vi "XDataNode8_6To8_5.vi"(10 "Version-State Cluster In":T1, 11 "XRef":refnum<vi>) -> (0 "Custom Label":string, 1 "Custom Warning To Issue":string, 2 "Version-State Cluster Out":T1, 3 "Action":T2)   [LabVIEW 2020]
uses:
  <vilib>/XSFPSupport/SFPChangeStateAction.ctl
  <vilib>/XNodeSupport/XNodeVersion.ctl
  <vilib>/XNodeSupport/XNodeUShort.ctl
  <vilib>/Platform/TimedLoop/XDataNode/XDataNode.ctl
  <vilib>/Platform/TimedLoop/XDataNode/timing_clust.ctl
  <vilib>/Platform/TimedLoop/XDataNode/nitl_modes.ctl
  <vilib>/Platform/TimedLoop/XDataNode/wakeup.ctl
  <vilib>/Platform/TimedLoop/XDataNode/TermInfo.ctl
  <vilib>/Platform/TimedLoop/XDataNode/nitl_TargetSpecificData.ctl
  <vilib>/Platform/TimedLoop/XDataNode/DN_Type.ctl
  <vilib>/Platform/TimedLoop/XDataNode/XDataNode8_5_0_1.ctl
  <vilib>/XSFPSupport/NI_XSFPSupport.lvlib
  <vilib>/XNodeSupport/NI_XNodeSupport.lvlib
  <vilib>/Platform/TimedLoop/XDataNode/XDataNode.xnode
  <vilib>/Platform/TimedLoop/XDataNode/XDNodeRunTimeDep.lvlib
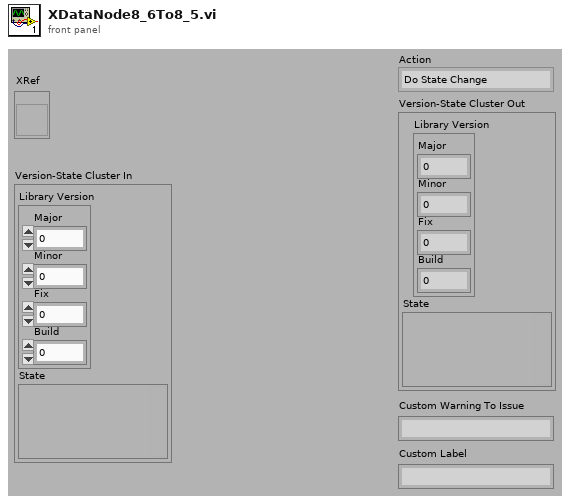
[diagram p1: front panel]
types:
  T1 = cluster{"Library Version":cluster{"Major":u16, "Minor":u16, "Fix":u16, "Build":u16}, "State":variant}
  T2 = typedef "NI_XSFPSupport.lvlib/SFPChangeStateAction.ctl" = enum32{"Do State Change", "Replace With Label", "Fail SFP"}
  T3 = typedef "XDataNode.xnode/XDataNode8_5_0_1.ctl" = cluster{"Timing":cluster{"Expected End [f-1]":u64, "Actual End [f-1]":u64, "Finished Late? [f-1]":bool, "Expected End [i-1]":u64, "Actual End [i-1]":u64, "Finished Late? [i-1]":bool, "Expected Start [i]":u64, "Actual Start [i]":u64, "Expected Start [f]":u64, "Actual Start [f]":u64, "Source Name":string, "Name":string, "Period":i64, "Deadline":i64, "Offset":i64, "Start":i64, "Priority":i32, "Timeout":i32, "Mode":T4, "Wakeup Reason":T5, "Error":errorcluster, "Source Type":string, "Secondary Source Type":string, "Global End Time":u64, "Global Start Time":u64, "Frame Duration":u64, "Iteration Duration":u64, "Assigned CPU":i32}, "Size":T6[], "Hidden":T6[], "Invisible":bool[], "Input?":bool, "timing src wired?":bool, "Target Specific Data":T7[], "G Only Data":variant, "DataNode_Type":T8}
  T4 = typedef "XDNodeRunTimeDep.lvlib/nitl_modes.ctl" = enum32{"No Change", "Process missed periods, maintain original phase", "Discard missed periods, maintain original phase", "Process missed periods, ignore original phase", "Discard missed periods, ignore original phase"}
  T5 = typedef "XDNodeRunTimeDep.lvlib/wakeup.ctl" = enum32{"Normal", "Aborted", "Asynchronous wakeup", "Timing source error", "Timed loop error", "Timeout"}
  T6 = typedef "XDataNode.xnode/TermInfo.ctl" = cluster{"ID":i32, "Wired?":bool, "Type":variant, "Name":string, "Input?":bool, "StaticID":i32}
  T7 = typedef "XDataNode.xnode/nitl_TargetSpecificData.ctl" = cluster{"Target Name":string, "Target Data":variant}
  T8 = typedef "XDataNode.xnode/DN_Type.ctl" = enum32{"TL_Lft_Ear", "TL_Rt_Ear", "TL_Lft_Dn", "TL_Rt_Dn", "TS_Lft_Ear", "TS_Rt_Ear", "TS_1stFrame_Lft_Dn", "TS_Lft_Dn", "TS_LastFrame_Rt_Dn", "TS_Rt_Dn", "TL_TS_Lft_Ear", "TL_TS_Rt_Ear", "TL_TS_Lft_Dn", "TL_TS_Rt_Dn", "TL_TS_1stFrame_Lft_Dn", "TL_TS_LastFrame_Rt_Dn"}
  T9 = typedef "XDataNode.xnode/XDataNode.ctl" = cluster{"Timing":T10, "Size":T6[], "Hidden":T6[], "Invisible":bool[], "Input?":bool, "timing src wired?":bool, "Target Specific Data":T7[], "G Only Data":variant, "DataNode_Type":T8}
  T10 = typedef "XDNodeRunTimeDep.lvlib/timing_clust.ctl" = cluster{"Expected End [f-1]":u64, "Actual End [f-1]":u64, "Finished Late? [f-1]":bool, "Expected End [i-1]":u64, "Actual End [i-1]":u64, "Finished Late? [i-1]":bool, "Expected Start [i]":u64, "Actual Start [i]":u64, "Expected Start [f]":u64, "Actual Start [f]":u64, "Source Name":string, "Structure Name":string, "Period":i64, "Deadline":i64, "Offset":i64, "Start":i64, "Priority":i32, "Timeout":i32, "Mode":T4, "Wakeup Reason":T5, "Error":errorcluster, "Source Type":string, "Secondary Source Type":string, "Global End Time":u64, "Global Start Time":u64, "Frame Duration":u64, "Iteration Duration":u64, "Assigned CPU":i32, "I/O Scan Engine Mode":u32}
  T11 = typedef "NI_XNodeSupport.lvlib/XNodeVersion.ctl" = cluster{"Major":T12, "Minor":T12, "Fix":T12, "Build":T12}
  T12 = typedef "NI_XNodeSupport.lvlib/XNodeUShort.ctl" = u16
  T13 = cluster{"Major":u16, "Minor":u16, "Fix":u16, "Build":u16}
  T14 = cluster{"Expected End [f-1]":u64, "Actual End [f-1]":u64, "Finished Late? [f-1]":bool, "Expected End [i-1]":u64, "Actual End [i-1]":u64, "Finished Late? [i-1]":bool, "Expected Start [i]":u64, "Actual Start [i]":u64, "Expected Start [f]":u64, "Actual Start [f]":u64, "Source Name":string, "Name":string, "Period":i64, "Deadline":i64, "Offset":i64, "Start":i64, "Priority":i32, "Timeout":i32, "Mode":T4, "Wakeup Reason":T5, "Error":errorcluster, "Source Type":string, "Secondary Source Type":string, "Global End Time":u64, "Global Start Time":u64, "Frame Duration":u64, "Iteration Duration":u64, "Assigned CPU":i32}
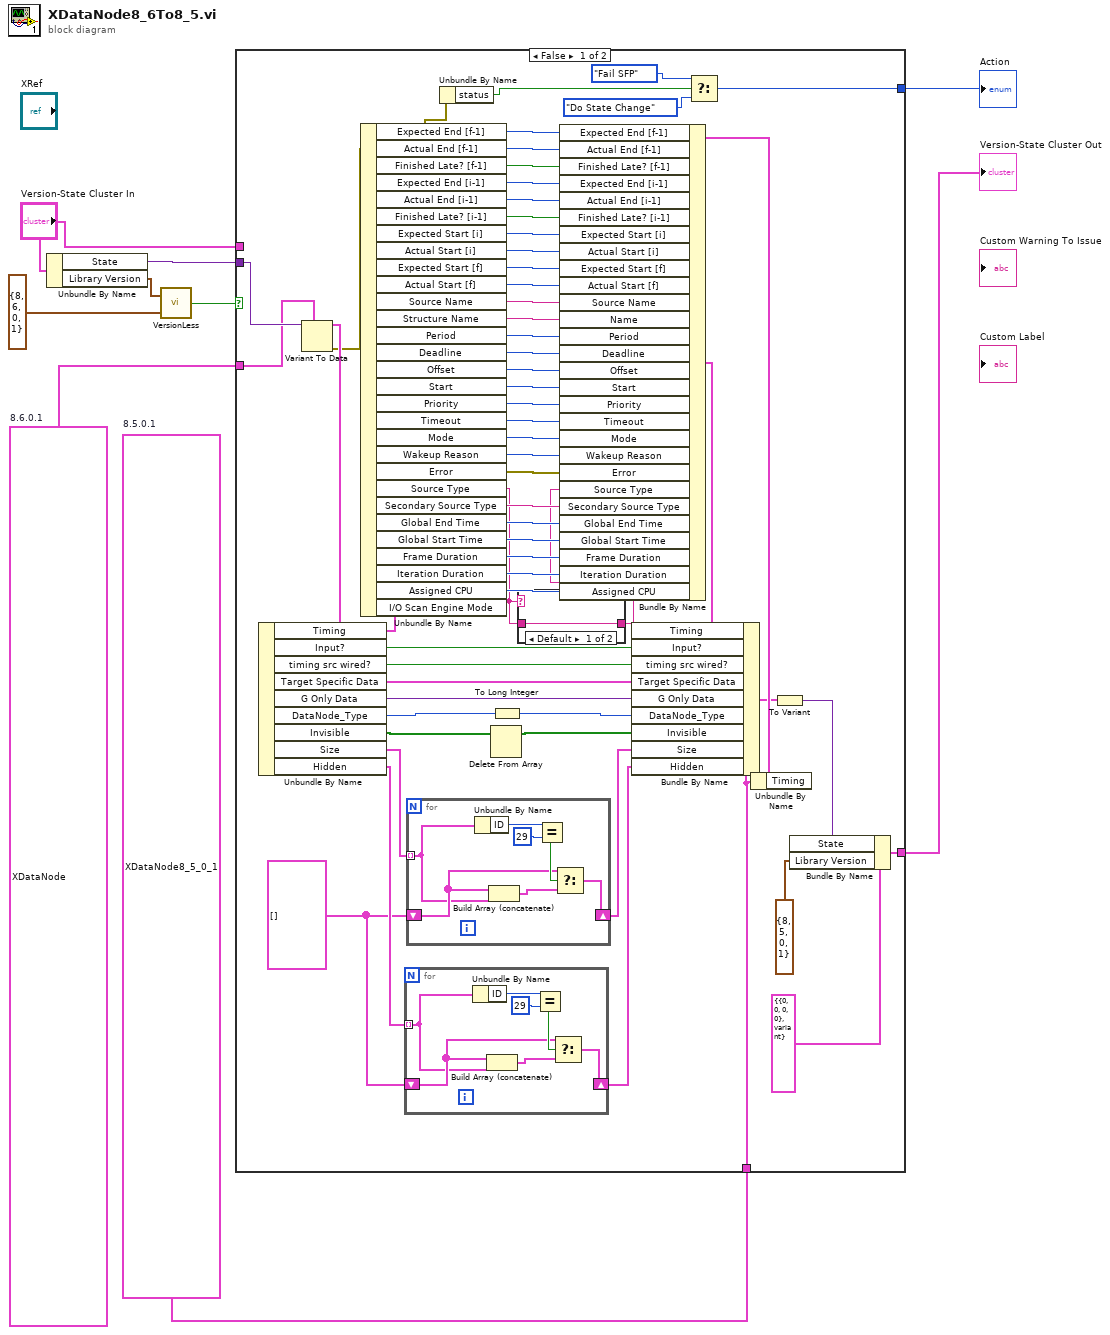
[diagram p0: block diagram]
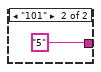
[diagram p2: hidden frame]
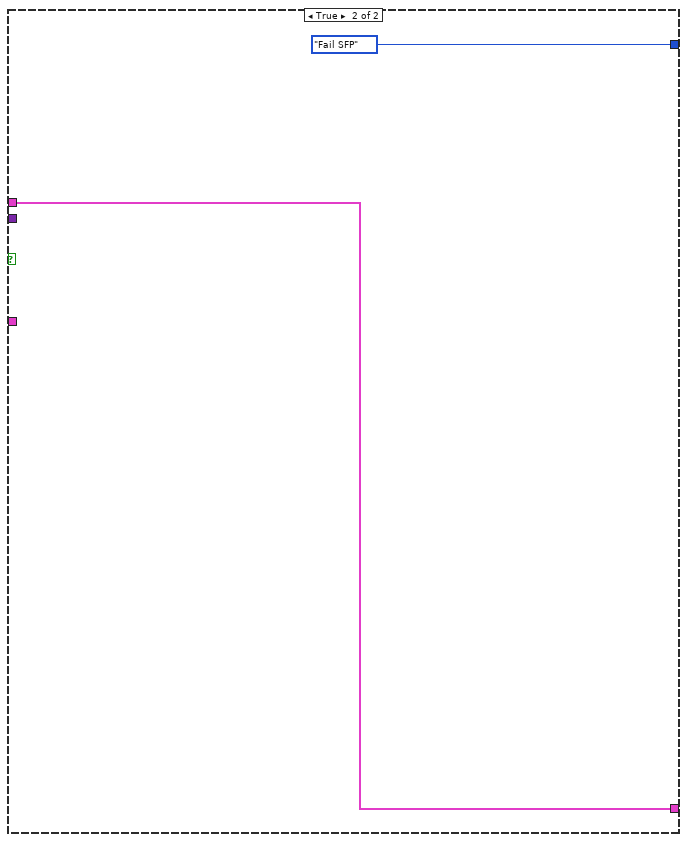
[diagram p3: hidden frame]
diagram:
  w3 = T3 {"Timing"={"Expected End [f-1]"=0, "Actual End [f-1]"=0, "Finished Late? [f-1]"=FALSE, "Expected End [i-1]"=0, "Actual End [i-1]"=0, "Finished Late? [i-1]"=FALSE, "Expected Start [i]"=0, "Actual Start [i]"=0, "Expected Start [f]"=0, "Actual Start [f]"=0, "Source Name"="", "Name"="", "Period"=0, "Deadline"=0, "Offset"=0, "Start"=0, "Priority"=0, "Timeout"=0, "Mode"=enum."No Change", "Wakeup Reason"=enum."Normal", "Error"={"status"=FALSE, "code"=0, "source"=""}, "Source Type"="", "Secondary Source Type"="", "Global End Time"=0, "Global Start Time"=0, "Frame Duration"=0, "Iteration Duration"=0, "Assigned CPU"=0}, "Size"=[], "Hidden"=[], "Invisible"=[], "Input?"=FALSE, "timing src wired?"=FALSE, "Target Specific Data"=[], "G Only Data"=variant, "DataNode_Type"=enum."TL_Lft_Ear"}  # 8.5.0.1
  w4 = T9 {"Timing"={"Expected End [f-1]"=0, "Actual End [f-1]"=0, "Finished Late? [f-1]"=FALSE, "Expected End [i-1]"=0, "Actual End [i-1]"=0, "Finished Late? [i-1]"=FALSE, "Expected Start [i]"=0, "Actual Start [i]"=0, "Expected Start [f]"=0, "Actual Start [f]"=0, "Source Name"="", "Structure Name"="", "Period"=0, "Deadline"=0, "Offset"=0, "Start"=0, "Priority"=0, "Timeout"=0, "Mode"=enum."No Change", "Wakeup Reason"=enum."Normal", "Error"={"status"=FALSE, "code"=0, "source"=""}, "Source Type"="", "Secondary Source Type"="", "Global End Time"=0, "Global Start Time"=0, "Frame Duration"=0, "Iteration Duration"=0, "Assigned CPU"=0, "I/O Scan Engine Mode"=0}, "Size"=[], "Hidden"=[], "Invisible"=[], "Input?"=FALSE, "timing src wired?"=FALSE, "Target Specific Data"=[], "G Only Data"=variant, "DataNode_Type"=enum."TL_Lft_Ear"}  # 8.6.0.1
  n1 = Unbundle By Name("Version-State Cluster In") -> ("State"=w5:variant, "Library Version"=w6:T13)
  n2 = call <vilib>:"VersionLess.vi"("y"=T11 {"Major"=8, "Minor"=6, "Fix"=0, "Build"=1}, "x"=w6) -> ("x < y?"=w8:bool)
  n3 = case shown="False" w8 {
    tunnel: [w18 SFPChangeStateAction."Fail SFP" ("Action")] -> w7
    tunnel: w5 -> [w68 _]
    tunnel: w4 -> [w67 _]
    tunnel: w3 -> [w64 _]
    tunnel: [w10 w85] -> w2
    tunnel: "Version-State Cluster In" -> [_ w85]
    frame False {
      w23 = T6[] [] ("Size")
      n4 = Variant To Data(type=w67, Variant=w68) -> (data=w66:T9, error out=w22:errorcluster)  [unwired: 1 in]
      n5 = Unbundle By Name(w66) -> ("Timing"=w65:T10, "Input?"=w35:bool, "timing src wired?"=w34:bool, "Target Specific Data"=w33:T7[], "G Only Data"=w32:variant, "DataNode_Type"=w31:T8, "Invisible"=w29:bool[], "Size"=w27:T6[], "Hidden"=w25:T6[])
      n6 = Unbundle By Name(w65) -> ("Expected End [f-1]"=w62:u64, "Actual End [f-1]"=w61:u64, "Finished Late? [f-1]"=w60:bool, "Expected End [i-1]"=w59:u64, "Actual End [i-1]"=w58:u64, "Finished Late? [i-1]"=w57:bool, "Expected Start [i]"=w56:u64, "Actual Start [i]"=w55:u64, "Expected Start [f]"=w54:u64, "Actual Start [f]"=w53:u64, "Source Name"=w52:string, "Structure Name"=w51:string, "Period"=w50:i64, "Deadline"=w49:i64, "Offset"=w48:i64, "Start"=w47:i64, "Priority"=w46:i32, "Timeout"=w45:i32, "Mode"=w44:T4, "Wakeup Reason"=w43:T5, "Error"=w42:errorcluster, "Source Type"=w15:string, "Secondary Source Type"=w41:string, "Global End Time"=w40:u64, "Global Start Time"=w39:u64, "Frame Duration"=w38:u64, "Iteration Duration"=w37:u64, "Assigned CPU"=w17:i32)  [unwired: 1 out]
      n7 = for {
        tunnel: w25 -> [w73] mode=indexing
        shift-right: [w71] -> w24
        shift-left: w23 -> [w74]
        n8 = Unbundle By Name(w73) -> ("ID"=w77:i32)
        n9 = Build Array (concatenate)(w74, w73) -> (w72:T6[])
        n10 = Equal?(x=w77, y=29) -> (x = y?=w75:bool)
        n11 = Select(t=w74, s=w75, f=w72) -> (s? t:f=w71:T6[])
      }
      n12 = for {
        tunnel: w27 -> [w80] mode=indexing
        shift-right: [w78] -> w26
        shift-left: w23 -> [w81]
        n13 = Unbundle By Name(w80) -> ("ID"=w84:i32)
        n14 = Build Array (concatenate)(w81, w80) -> (w79:T6[])
        n15 = Equal?(x=w84, y=29) -> (x = y?=w82:bool)
        n16 = Select(t=w81, s=w82, f=w79) -> (s? t:f=w78:T6[])
      }
      n17 = Unbundle By Name(w22) -> ("status"=w21:bool)
      n18 = Delete From Array(array=w29) -> (array with subset deleted=w28:bool[])  [unwired: 2 in, 1 out]
      n19 = To Long Integer(number=w31) -> (32bit integer=w30:i32)
      n20 = case shown="Default" w15 {
        tunnel: [w69 "5"] -> w16
        tunnel: w15 -> [w69 _]
        frame Default {
        }
        frame "101" {
        }
      }
      n21 = Select(t=SFPChangeStateAction."Fail SFP" ("Action"), s=w21, f=SFPChangeStateAction."Do State Change" ("Action")) -> (s? t:f=w18:T2)
      n22 = Unbundle By Name(w64) -> ("Timing"=w63:T14)
      n23 = Bundle By Name(cluster=w63, "Expected End [f-1]"=w62, "Actual End [f-1]"=w61, "Finished Late? [f-1]"=w60, "Expected End [i-1]"=w59, "Actual End [i-1]"=w58, "Finished Late? [i-1]"=w57, "Expected Start [i]"=w56, "Actual Start [i]"=w55, "Expected Start [f]"=w54, "Actual Start [f]"=w53, "Source Name"=w52, "Name"=w51, "Period"=w50, "Deadline"=w49, "Offset"=w48, "Start"=w47, "Priority"=w46, "Timeout"=w45, "Mode"=w44, "Wakeup Reason"=w43, "Error"=w42, "Source Type"=w16, "Secondary Source Type"=w41, "Global End Time"=w40, "Global Start Time"=w39, "Frame Duration"=w38, "Iteration Duration"=w37, "Assigned CPU"=w17) -> (w36:T14)
      n24 = Bundle By Name(cluster=w64, "Timing"=w36, "Input?"=w35, "timing src wired?"=w34, "Target Specific Data"=w33, "G Only Data"=w32, "DataNode_Type"=w30, "Invisible"=w28, "Size"=w26, "Hidden"=w24) -> (w14:T3)
      n25 = To Variant(anything=w14) -> (Variant=w11:variant)
      n26 = Bundle By Name(cluster=T1 {"Library Version"={"Major"=0, "Minor"=0, "Fix"=0, "Build"=0}, "State"=variant} ("Version-State Cluster Out"), "State"=w11, "Library Version"=T11 {"Major"=8, "Minor"=5, "Fix"=0, "Build"=1} ("y")) -> (w10:T1)
    }
    frame True {
    }
  }
  "Action" <- w7
  "Version-State Cluster Out" <- w2
